vi "Get PDC Real Data.vi"(7 "Initialize Time":bool, 11 "Pseudo PDC ID":i32) -> (0 "PDC Real Data":T1, 1 "Number of PMUs":i32, 2 "Time Stamp":timestamp, 3 "Data OK":bool, 4 "Relative System Clock (ms)":dbl, 6 "dt (ms)":dbl)   [LabVIEW 2013, in "PMU Recorder Light.lvlib" / "Statnett C37.118 DLL.lvclass"]
uses:
  Statnett C37.118 DLL.lvclass
  <vilib>/Utility/miscctls.llb/LVDateTimeRec.ctl
  c37118-dll/C37118-DLL.lvlib
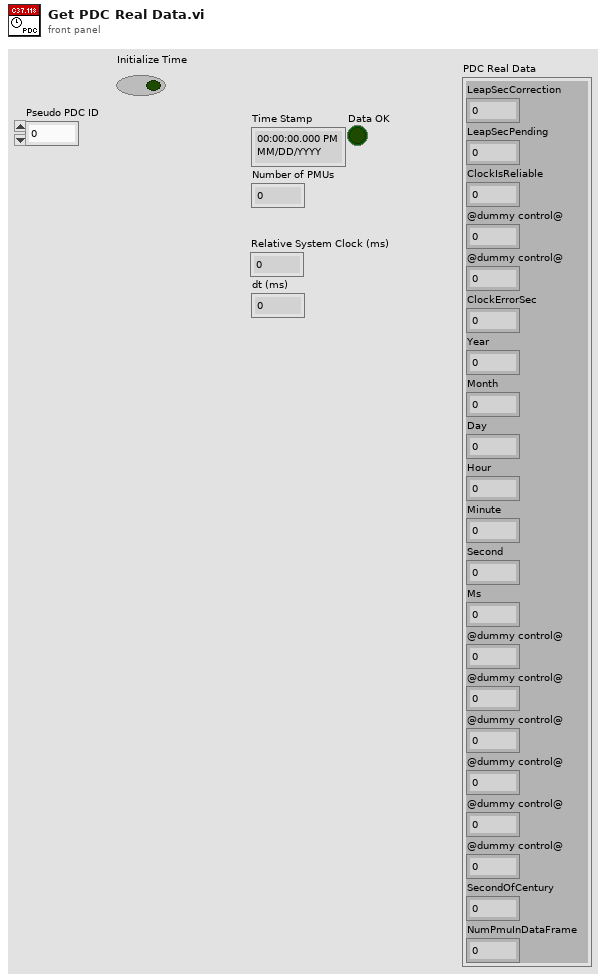
[diagram p1: front panel]
types:
  T1 = cluster{"LeapSecCorrection":i32, "LeapSecPending":u8, "ClockIsReliable":u8, "@dummy control@":i8, "@dummy control@":i8, "ClockErrorSec":sgl, "Year":i16, "Month":i16, "Day":i16, "Hour":i16, "Minute":i16, "Second":i16, "Ms":i16, "@dummy control@":i8, "@dummy control@":i8, "@dummy control@":i8, "@dummy control@":i8, "@dummy control@":i8, "@dummy control@":i8, "SecondOfCentury":dbl, "NumPmuInDataFrame":i32}
  T2 = typedef "LVDateTimeRec.ctl" = cluster{"fractional second":dbl, "second":i32, "minute":i32, "hour":i32, "day of month":i32, "month":i32, "year":i32, "day of week":i32, "day of year":i32, "DST":i32}
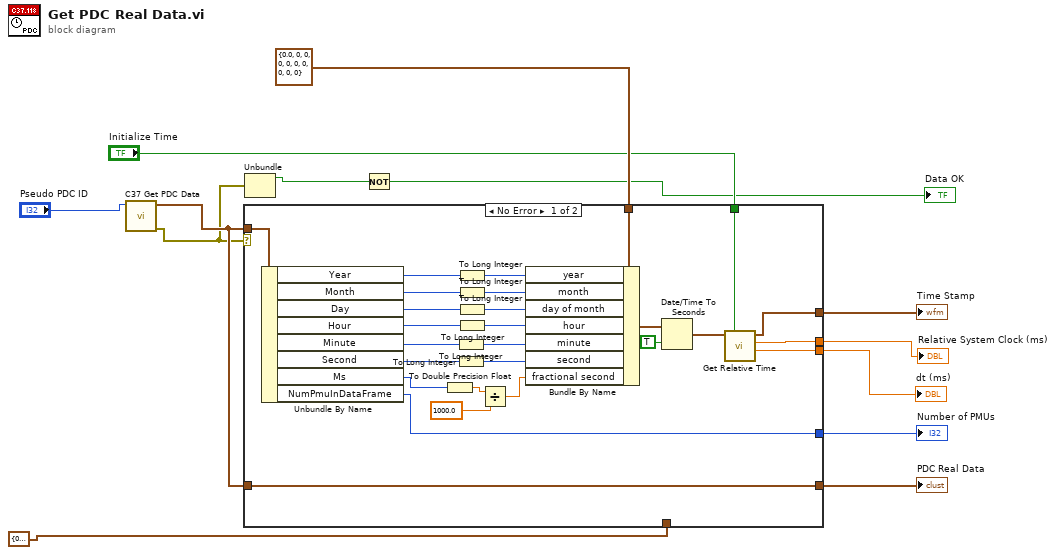
[diagram p0: block diagram]
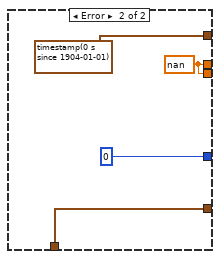
[diagram p2: hidden frame]
diagram:
  n1 = call "C37 Get PDC Data.vi"("Pseudo PDC ID"="Pseudo PDC ID") -> ("error out"=w3:errorcluster, "PDC Data"=w4:T1)  [unwired: 9 in]
  n2 = case shown="No Error" w3 {
    tunnel: w4 -> [w40 _]
    tunnel: T2 {"fractional second"=0.0, "second"=0, "minute"=0, "hour"=0, "day of month"=0, "month"=0, "year"=0, "day of week"=0, "day of year"=0, "DST"=0} ("date time rec") -> [w39 _]
    tunnel: [w21 0 ("NumPmuInDataFrame")] -> w11
    tunnel: [w18 timestamp(0 s since 1904-01-01) ("time stamp")] -> w12
    tunnel: w4 -> [w20 _]
    tunnel: [w20 w42] -> w9
    tunnel: T1 {"LeapSecCorrection"=0, "LeapSecPending"=0, "ClockIsReliable"=0, "@dummy control@"=0, "@dummy control@"=0, "ClockErrorSec"=0.0, "Year"=0, "Month"=0, "Day"=0, "Hour"=0, "Minute"=0, "Second"=0, "Ms"=0, "@dummy control@"=0, "@dummy control@"=0, "@dummy control@"=0, "@dummy control@"=0, "@dummy control@"=0, "@dummy control@"=0, "SecondOfCentury"=0.0, "NumPmuInDataFrame"=0} ("rd out") -> [_ w42]
    tunnel: [w17 w41] -> w8
    tunnel: [w16 w41] -> w7
    tunnel: "Initialize Time" -> [w15 _]
    frame No Error {
      n3 = Unbundle By Name(w40) -> ("Year"=w38:i16, "Month"=w36:i16, "Day"=w34:i16, "Hour"=w32:i16, "Minute"=w30:i16, "Second"=w28:i16, "Ms"=w26:i16, "NumPmuInDataFrame"=w21:i32)
      n4 = To Double Precision Float(number=w26) -> (double precision float=w25:dbl)
      n5 = To Long Integer(number=w30) -> (32bit integer=w29:i32)
      n6 = To Long Integer(number=w28) -> (32bit integer=w27:i32)
      n7 = To Long Integer(number=w38) -> (32bit integer=w37:i32)
      n8 = To Long Integer(number=w36) -> (32bit integer=w35:i32)
      n9 = To Long Integer(number=w34) -> (32bit integer=w33:i32)
      n10 = To Long Integer(number=w32) -> (32bit integer=w31:i32)
      n11 = Divide(x=w25, y=1000.0) -> (x/y=w23:dbl)
      n12 = Bundle By Name(cluster=w39, "year"=w37, "month"=w35, "day of month"=w33, "hour"=w31, "minute"=w29, "second"=w27, "fractional second"=w23) -> (w22:T2)
      n13 = Date/Time To Seconds(1:TRUE ("is UTC (F)"), 2:w22) -> (0:w19:timestamp)
      n14 = call "Get Relative Time.vi"("Init?"=w15, "Time Stamp In"=w19) -> ("dt (ms)"=w17:dbl, "Relative System Clock (ms)"=w16:dbl, "Time Stamp Out"=w18:timestamp)  [unwired: 7 in]
    }
    frame Error {
      w41 = nan ("Relative System Clock (ms)")
    }
  }
  "Time Stamp" <- w12
  "Number of PMUs" <- w11
  "PDC Real Data" <- w9
  "Relative System Clock (ms)" <- w7
  "dt (ms)" <- w8
  n15 = Unbundle(w3) -> ("status"=w2:bool)  [unwired: 2 out]
  n16 = Not(x=w2) -> (.not. x?=→"Data OK":bool)
